vi "Template.vi"(8 "error in (no error)":errorcluster, 10 "Response String in":string, 11 "Return Request in":T1) -> (0 "error out":errorcluster, 2 "Response String out":string, 3 "Return Request out":T1)   [LabVIEW 2017]
uses:
  Libraries/SSH/Return Request Configuration.ctl
  Libraries/SSH/Response Configuration.ctl
  Libraries/SSH/SSH.lvlib
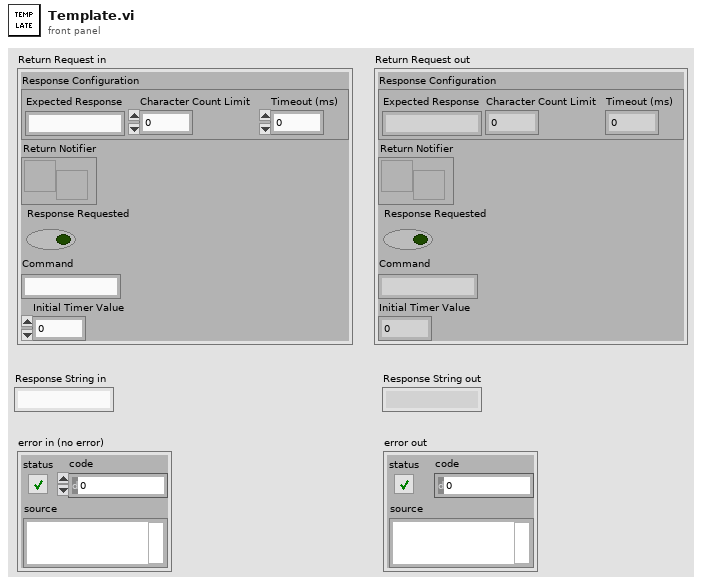
[diagram p1: front panel]
types:
  T1 = typedef "SSH.lvlib/Return Request Configuration.ctl" = cluster{"Response Configuration":T2, "Return Notifier":refnum<notifier>, "Response Requested":bool, "Command":string, "Initial Timer Value":u32}
  T2 = typedef "SSH.lvlib/Response Configuration.ctl" = cluster{"Expected Response":string, "Character Count Limit":i32, "Timeout (ms)":u32}
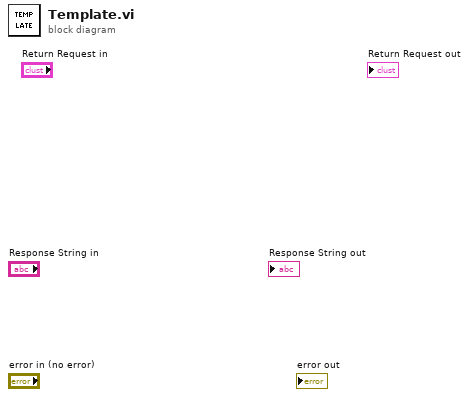
[diagram p0: block diagram]
diagram:
